vi "Init.vi"(8 "error in (no error)":errorcluster, 11 "SolarSystems M266 in":refnum<class "SolarSystems M266.lvclass">) -> (0 "error out":errorcluster, 3 "SolarSystems M266 out":refnum<class "SolarSystems M266.lvclass">)   [LabVIEW 2014, in "SolarSystems M266.lvclass"]
uses:
  SolarSystems M266.lvclass
  Framework/Hardware/ParameterDevice/ParameterDevice.lvclass
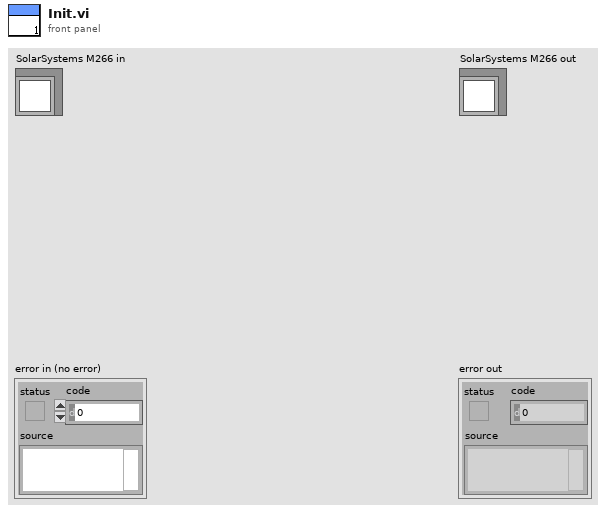
[diagram p1: front panel]
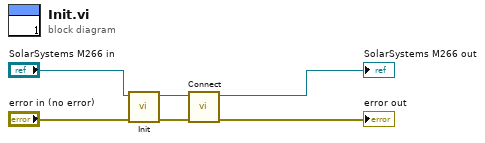
[diagram p0: block diagram]
diagram:
  n1 = call-parent "Init.vi"("error in (no error)"="error in (no error)", "Device in"="SolarSystems M266 in") -> ("error out"=w3:errorcluster, "Device out"=w4:refnum<class "SolarSystems M266.lvclass">)  [unwired: 8 in]
  n2 = call-dynamic "Connect.vi"("error in (no error)"=w3, "SolarSystems M266 in"=w4) -> ("error out"=→"error out":errorcluster, "SolarSystems M266 out"=→"SolarSystems M266 out":refnum<class "SolarSystems M266.lvclass">)  [unwired: 8 in]
